vi "CRYAutosave run check.vi"(5 "filename option":enum16{"auto", "prompt"}(ring), 6 "save in":enum16{"Data", "Results", "Waveforms"}(ring), 7 "data format":u16, 8 "fn construction":i32[](array[numeric]), 9 "Autosave folder":path, 10 "Item Names":string[](array[string])) -> (2 "number":i32, 3 "save able?":bool)   [LabVIEW 2013]
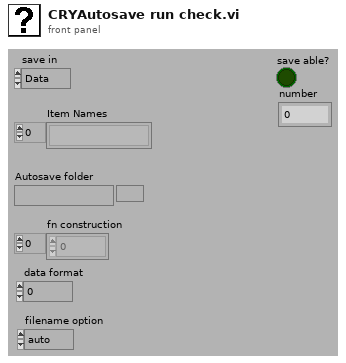
[diagram p1: front panel]
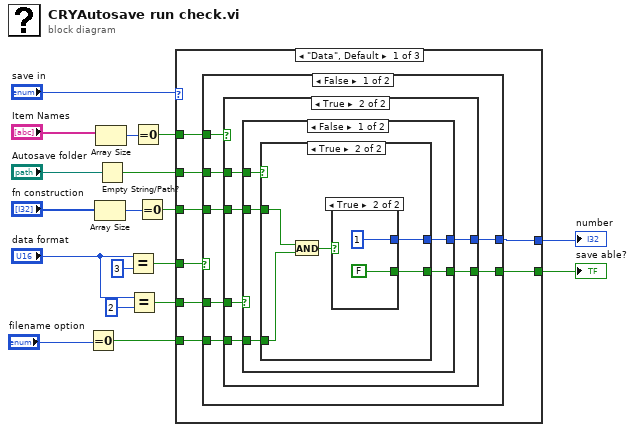
[diagram p0: block diagram]
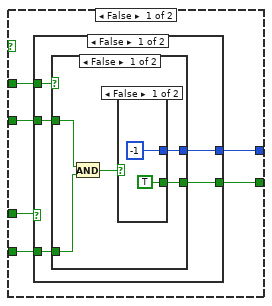
[diagram p2: hidden frame]
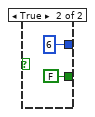
[diagram p3: hidden frame]
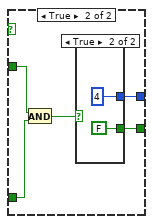
[diagram p4: hidden frame]
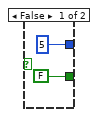
[diagram p5: hidden frame]
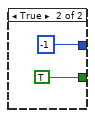
[diagram p6: hidden frame]
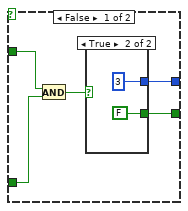
[diagram p7: hidden frame]
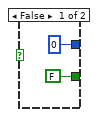
[diagram p8: hidden frame]
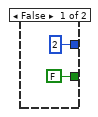
[diagram p9: hidden frame]
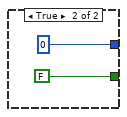
[diagram p10: hidden frame]
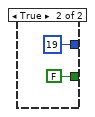
[diagram p11: hidden frame]
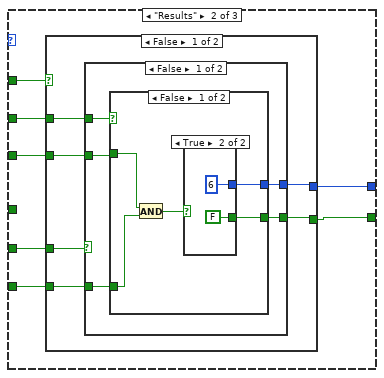
[diagram p12: hidden frame]
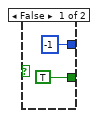
[diagram p13: hidden frame]
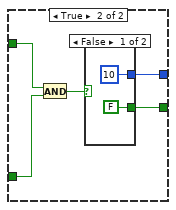
[diagram p14: hidden frame]
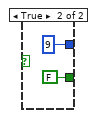
[diagram p15: hidden frame]
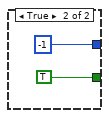
[diagram p16: hidden frame]
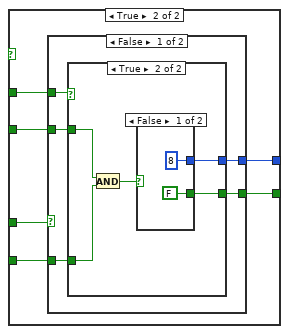
[diagram p17: hidden frame]
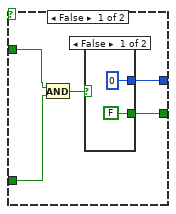
[diagram p18: hidden frame]
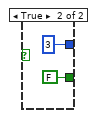
[diagram p19: hidden frame]
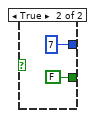
[diagram p20: hidden frame]
diagram:
  n1 = Equal To 0?(x="filename option") -> (x = 0?=w1:bool)
  n2 = Array Size(array="fn construction") -> (size(s)=w11:i32)
  n3 = Array Size(array="Item Names") -> (size(s)=w17:i32)
  n4 = Empty String/Path?(string/path="Autosave folder") -> (empty?=w13:bool)
  n5 = Equal?(x="data format", y=u16 3) -> (x = y?=w6:bool)
  n6 = Equal?(x="data format", y=u16 2) -> (x = y?=w3:bool)
  n7 = Equal To 0?(x=w17) -> (x = 0?=w15:bool)
  n8 = Equal To 0?(x=w11) -> (x = 0?=w10:bool)
  n9 = case shown="\"Data\", Default" "save in" {
    tunnel: w15 -> [w26 w99 w168]
    tunnel: w13 -> [w23 w98 w167]
    tunnel: w10 -> [w22 w102 w172]
    tunnel: [w25 w103 w170] -> w9
    tunnel: [w24 w104 w171] -> w8
    tunnel: w6 -> [w21 _ _]
    tunnel: w3 -> [w20 w101 _]
    tunnel: w1 -> [w19 w100 w169]
    frame "Data", Default {
      n10 = case shown="False" w21 {
        tunnel: w26 -> [w33 _]
        tunnel: [w32 FALSE] -> w25
        tunnel: [w31 19 ("y")] -> w24
        tunnel: w23 -> [w30 _]
        tunnel: w22 -> [w29 _]
        tunnel: w20 -> [w28 _]
        tunnel: w19 -> [w27 _]
        frame False {
          n11 = case shown="True" w33 {
            tunnel: w30 -> [w39 w70]
            tunnel: w29 -> [w38 w69]
            tunnel: [w37 w68] -> w31
            tunnel: [w36 w67] -> w32
            tunnel: w28 -> [w35 w66]
            tunnel: w27 -> [w34 w65]
            frame False {
              n12 = case shown="False" w35 {
                tunnel: w39 -> [w44 _]
                tunnel: w38 -> [w43 _]
                tunnel: [w42 -1] -> w37
                tunnel: [w41 TRUE] -> w36
                tunnel: w34 -> [w40 _]
                frame False {
                  n13 = case shown="False" w44 {
                    tunnel: w43 -> [w47 w56]
                    tunnel: [w49 w58] -> w42
                    tunnel: [w48 w57] -> w41
                    tunnel: w40 -> [w46 w55]
                    frame False {
                      n14 = And(x=w47, y=w46) -> (x .and. y?=w45:bool)
                      n15 = case shown="False" w45 {
                        tunnel: [-1 ("y") 6 ("y")] -> w49
                        tunnel: [TRUE FALSE] -> w48
                        frame False {
                        }
                        frame True {
                        }
                      }
                    }
                    frame True {
                      n16 = And(x=w56, y=w55) -> (x .and. y?=w54:bool)
                      n17 = case shown="True" w54 {
                        tunnel: [5 ("y") 4 ("y")] -> w58
                        tunnel: [FALSE FALSE] -> w57
                        frame False {
                        }
                        frame True {
                        }
                      }
                    }
                  }
                }
                frame True {
                }
              }
            }
            frame True {
              n18 = case shown="False" w66 {
                tunnel: w70 -> [w75 _]
                tunnel: w69 -> [w74 _]
                tunnel: [w73 0 ("y")] -> w68
                tunnel: [w72 FALSE] -> w67
                tunnel: w65 -> [w71 _]
                frame False {
                  n19 = case shown="True" w75 {
                    tunnel: w74 -> [w78 w86]
                    tunnel: [w80 w89] -> w73
                    tunnel: [w79 w88] -> w72
                    tunnel: w71 -> [w77 w87]
                    frame False {
                      n20 = And(x=w78, y=w77) -> (x .and. y?=w76:bool)
                      n21 = case shown="True" w76 {
                        tunnel: [0 ("y") 3 ("y")] -> w80
                        tunnel: [FALSE FALSE] -> w79
                        frame False {
                        }
                        frame True {
                        }
                      }
                    }
                    frame True {
                      n22 = And(x=w86, y=w87) -> (x .and. y?=w85:bool)
                      n23 = case shown="True" w85 {
                        tunnel: [2 ("y") 1 ("y")] -> w89
                        tunnel: [FALSE FALSE] -> w88
                        frame False {
                        }
                        frame True {
                        }
                      }
                    }
                  }
                }
                frame True {
                }
              }
            }
          }
        }
        frame True {
        }
      }
    }
    frame "Results" {
      n24 = case shown="False" w99 {
        tunnel: w98 -> [w110 w141]
        tunnel: w102 -> [w109 w140]
        tunnel: [w107 w139] -> w103
        tunnel: [w108 w138] -> w104
        tunnel: w101 -> [w106 w137]
        tunnel: w100 -> [w105 w136]
        frame False {
          n25 = case shown="False" w106 {
            tunnel: w110 -> [w115 _]
            tunnel: w109 -> [w114 _]
            tunnel: [w113 -1 ("y")] -> w108
            tunnel: [w112 TRUE] -> w107
            tunnel: w105 -> [w111 _]
            frame False {
              n26 = case shown="False" w115 {
                tunnel: w114 -> [w118 w126]
                tunnel: [w120 w129] -> w112
                tunnel: [w119 w128] -> w113
                tunnel: w111 -> [w117 w127]
                frame False {
                  n27 = And(x=w118, y=w117) -> (x .and. y?=w116:bool)
                  n28 = case shown="True" w116 {
                    tunnel: [TRUE FALSE] -> w120
                    tunnel: [-1 ("y") 6 ("y")] -> w119
                    frame False {
                    }
                    frame True {
                    }
                  }
                }
                frame True {
                  n29 = And(x=w126, y=w127) -> (x .and. y?=w125:bool)
                  n30 = case shown="False" w125 {
                    tunnel: [FALSE FALSE] -> w129
                    tunnel: [10 ("y") 9 ("y")] -> w128
                    frame False {
                    }
                    frame True {
                    }
                  }
                }
              }
            }
            frame True {
            }
          }
        }
        frame True {
          n31 = case shown="False" w137 {
            tunnel: w141 -> [w146 _]
            tunnel: w140 -> [w145 _]
            tunnel: [w144 FALSE] -> w139
            tunnel: [w143 0 ("y")] -> w138
            tunnel: w136 -> [w142 _]
            frame False {
              n32 = case shown="True" w146 {
                tunnel: w145 -> [w149 w158]
                tunnel: [w151 w160] -> w144
                tunnel: [w150 w159] -> w143
                tunnel: w142 -> [w148 w157]
                frame False {
                  n33 = And(x=w149, y=w148) -> (x .and. y?=w147:bool)
                  n34 = case shown="False" w147 {
                    tunnel: [FALSE FALSE] -> w151
                    tunnel: [0 ("y") 3 ("y")] -> w150
                    frame False {
                    }
                    frame True {
                    }
                  }
                }
                frame True {
                  n35 = And(x=w158, y=w157) -> (x .and. y?=w156:bool)
                  n36 = case shown="False" w156 {
                    tunnel: [FALSE FALSE] -> w160
                    tunnel: [8 ("y") 7 ("y")] -> w159
                    frame False {
                    }
                    frame True {
                    }
                  }
                }
              }
            }
            frame True {
            }
          }
        }
      }
    }
    frame "Waveforms" {
      n37 = case shown="False" w168 {
        tunnel: w167 -> [w177 w200]
        tunnel: w172 -> [w176 w199]
        tunnel: [w175 w198] -> w171
        tunnel: [w174 w197] -> w170
        tunnel: w169 -> [w173 w196]
        frame False {
          n38 = case shown="True" w177 {
            tunnel: w176 -> [w180 w189]
            tunnel: [w182 w191] -> w175
            tunnel: [w181 w190] -> w174
            tunnel: w173 -> [w179 w188]
            frame False {
              n39 = And(x=w180, y=w179) -> (x .and. y?=w178:bool)
              n40 = case shown="True" w178 {
                tunnel: [-1 ("y") 6 ("y")] -> w182
                tunnel: [TRUE FALSE] -> w181
                frame False {
                }
                frame True {
                }
              }
            }
            frame True {
              n41 = And(x=w189, y=w188) -> (x .and. y?=w187:bool)
              n42 = case shown="False" w187 {
                tunnel: [18 ("y") 17 ("y")] -> w191
                tunnel: [FALSE FALSE] -> w190
                frame False {
                }
                frame True {
                }
              }
            }
          }
        }
        frame True {
          n43 = case shown="False" w200 {
            tunnel: w199 -> [w203 w212]
            tunnel: [w205 w214] -> w198
            tunnel: [w204 w213] -> w197
            tunnel: w196 -> [w202 w211]
            frame False {
              n44 = And(x=w203, y=w202) -> (x .and. y?=w201:bool)
              n45 = case shown="False" w201 {
                tunnel: [0 ("y") 3 ("y")] -> w205
                tunnel: [FALSE FALSE] -> w204
                frame False {
                }
                frame True {
                }
              }
            }
            frame True {
              n46 = And(x=w212, y=w211) -> (x .and. y?=w210:bool)
              n47 = case shown="False" w210 {
                tunnel: [16 ("y") 15 ("y")] -> w214
                tunnel: [FALSE FALSE] -> w213
                frame False {
                }
                frame True {
                }
              }
            }
          }
        }
      }
    }
  }
  "save able?" <- w9
  "number" <- w8
